vi "Zaber A Series Commands and Responses.vi"() -> ()   [LabVIEW 2018]
doc: "This is a basic example demonstrating some of the low-level read and write VIs, with some example commands and a variety of output formats displayed."
uses:
  Zaber A Series.lvlib
panel:
  in  "Command":string
  out "Response Bundle Array":T1(array[cluster])
  out "First Response Data Value":string
  out "First Response Device Number":string
  out "Response String Array":string[](array[string])
  in  "VISA resource name":refnum<visa-resource-name>
  # "(c) 2017-2020 Zaber Technologies.  ALL RIGHTS RESERVED."
  # "The purpose of this example is to show how you can enter commands and read back\nresponses. There are a number of ways to read responses, whether you just read one \nresponse, only want want part of the response, or prefer the complete string. Try writing\nsome of the example commands and see what response options are available. \n\nEnter the VISA resource your device is connected to and the Command string before running the VI."
  # "Example commands: \n'home' - device retracts to find the reference position\n'move rel 5000' - move the device by 5000 microsteps\n'01 get maxspeed' - returns the movement speed setting for device 1"
  # "If the command or data value you supply is not valid, you will get a warning message with a description of what the problem\nis in the error output."
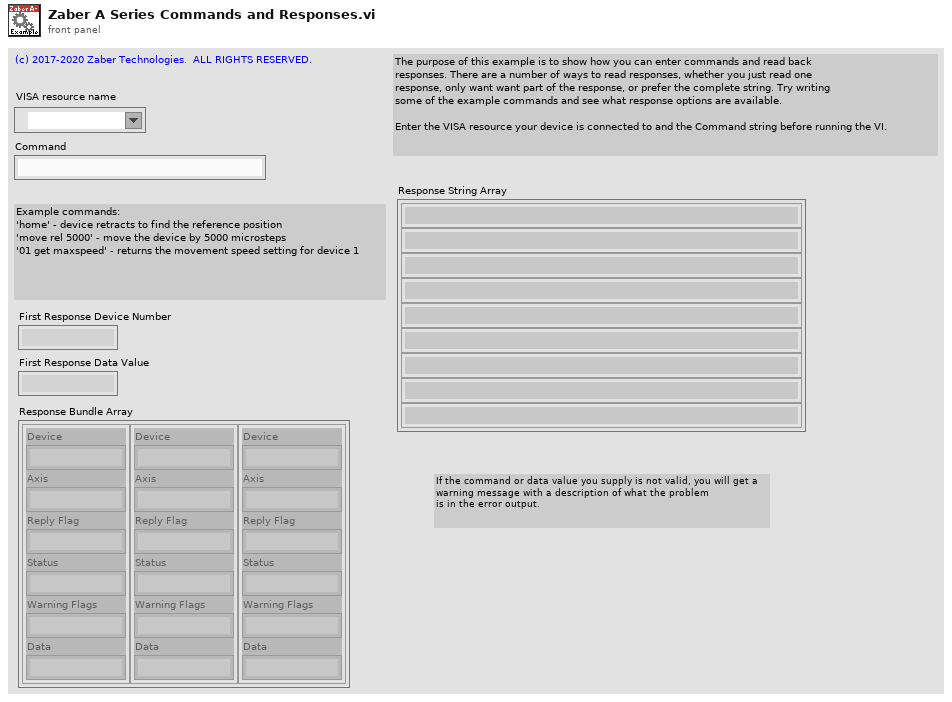
[diagram p1: front panel]
types:
  T1 = cluster{"Device":string, "Axis":string, "Reply Flag":string, "Status":string, "Warning Flags":string, "Data":string}[]
  T2 = cluster{"Device":string, "Axis":string, "Reply Flag":string, "Status":string, "Warning Flags":string, "Data":string}
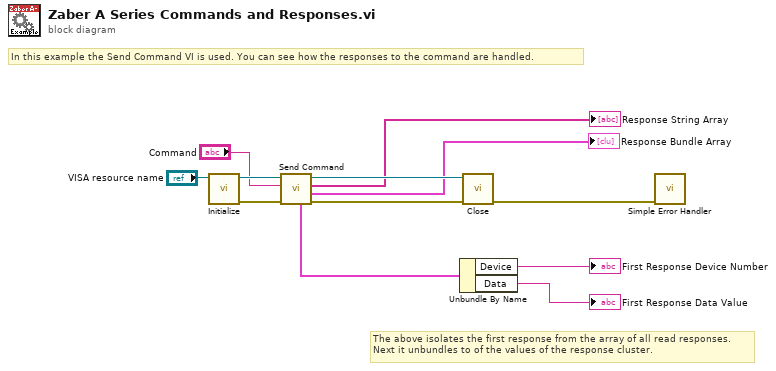
[diagram p0: block diagram]
diagram:
  # "In this example the Send Command VI is used. You can see how the responses to the command are handled."
  # "The above isolates the first response from the array of all read responses.\nNext it unbundles to of the values of the response cluster."
  n1 = call "Initialize.vi"("VISA resource name"="VISA resource name") -> ("error out"=w7:errorcluster, "VISA resource name out"=w8:refnum<visa-resource-name>)  [unwired: 9 in]
  n2 = call "Send Command.vi"("error in (no error)"=w7, "Command"="Command", "VISA resource name"=w8) -> ("error out"=w6:errorcluster, "Response Bundle Array"=→"Response Bundle Array":T1, "Response String Array"=→"Response String Array":string[], "VISA resource name out"=w5:refnum<visa-resource-name>, "First Response Bundle"=w1:T2)  [unwired: 3 in, 1 out]
  n3 = Unbundle By Name(w1) -> ("Device"=→"First Response Device Number":string, "Data"=→"First Response Data Value":string)
  n4 = call "Close.vi"("error in (no error)"=w6, "VISA resource name"=w5) -> ("error out"=w9:errorcluster)  [unwired: 9 in]
  n5 = call <vilib>:"Simple Error Handler.vi"("error in (no error)"=w9) -> ()  [unwired: 4 in, 5 out]
